vi "Periodic Tasks.vi"   [LabVIEW 2020]
doc: "This VI runs in parallel to other tasks. It can contain as many user-defined periodic loops as you need. These can carry out PID or other sorts of timed response."
uses:
  <vilib>/Rock Robotics/WPI/ThirdParty/JAS_Junk/TrajLib/PIDController_AtSetpoint.vi
  <vilib>/Rock Robotics/WPI/ThirdParty/JAS_Junk/TrajLib/PIDController_SetPIDF.vi
  <vilib>/Rock Robotics/WPI/ThirdParty/JAS_Junk/TrajLib/PIDController_SetDerivativeFilter.vi
  <vilib>/Rock Robotics/WPI/ThirdParty/JAS_Junk/TrajLib/PIDController_SetIntegratorRange.vi
  <vilib>/Rock Robotics/WPI/ThirdParty/JAS_Junk/TrajLib/PIDController_SetTolerancePandV.vi
  <vilib>/Rock Robotics/WPI/ThirdParty/JAS_Junk/TrajLib/PIDController_DisableContinousInput.vi
  <vilib>/Rock Robotics/WPI/ThirdParty/JAS_Junk/TrajLib/PIDController_EnableContinousInput.vi
  <vilib>/Rock Robotics/WPI/ThirdParty/JAS_Junk/TrajLib/PIDController_Reset.vi
  <vilib>/Rock Robotics/WPI/ThirdParty/JAS_Junk/TrajLib/PIDController_New.vi
  <vilib>/Rock Robotics/WPI/ThirdParty/JAS_Junk/TrajLib/PIDController_SetOutputLimits.vi
  <vilib>/Rock Robotics/WPI/ThirdParty/JAS_Junk/TrajLib/PIDController_NewPeriod.vi
  <vilib>/Rock Robotics/SystemInterfaces/NetworkCommunication/NetComm_UsageReport_report.vi
  Robot Global Data.vi
  <vilib>/Rock Robotics/WPI/ThirdParty/JAS_Junk/TrajLib/Util_LibraryGlobals.vi
  <vilib>/Rock Robotics/WPI/ThirdParty/JAS_Junk/TrajLib/PIDController_AdvCalculate_FF_Sp_Pv.vi
  <vilib>/Rock Robotics/WPI/ThirdParty/JAS_Junk/TrajLib/Trajectory_Library.lvlib
types:
  T1 = typedef "WPI_MotorControlDeviceRef.ctl" = cluster{"DeviceStatus":errorcluster, "Type":T2, "PWM":cluster{"PWM Channel":T3, "DeadBand":T4}, "CAN":cluster{"Device Number":u8, "SetOutput VI Ref":variant, "GetOutput VI Ref":variant, "Enable VI Ref":variant, "Disable VI Ref":variant, "Data":variant}, "Invert":bool, "DIO PWM":cluster{"PWM \"Enable\" Channel":T3, "DIOChannel":T5, "PWM Rate":dbl}}
  T2 = typedef "WPI_MotorControlType.ctl" = enum16{"PWM", "CAN", "DIO PWM"}
  T3 = typedef "FPGA_DIOPWMChannel.ctl" = enum8{"PWM 0", "PWM 1", "PWM 2", "PWM 3", "PWM 4", "PWM 5", "PWM 6", "PWM 7", "PWM 8", "PWM 9", "PWM MXP 0", "PWM MXP 1", "PWM MXP 2", "PWM MXP 3", "PWM MXP 4", "PWM MXP 5", "PWM MXP 6", "PWM MXP 7", "PWM MXP 8", "PWM MXP 9", "Invalid"}
  T4 = typedef "WPI_PWMDeadband.ctl" = cluster{"Name":string, "maxPositivePwm":i32, "minPositivePwm":i32, "centerPwm":i32, "maxNegativePwm":i32, "minNegativePwm":i32, "angularRange":u16}
  T5 = typedef "FPGA_DIOChannel.ctl" = enum8{"DIO 0", "DIO 1", "DIO 2", "DIO 3", "DIO 4", "DIO 5", "DIO 6", "DIO 7", "DIO 8", "DIO 9", "DIO MXP 0", "DIO MXP 1", "DIO MXP 2", "DIO MXP 3", "DIO MXP 4", "DIO MXP 5", "DIO MXP 6", "DIO MXP 7", "DIO MXP 8", "DIO MXP 9", "DIO MXP 10", "DIO MXP 11", "DIO MXP 12", "DIO MXP 13", "DIO MXP 14", "DIO MXP 15", "SPI Port CS1", "SPI Port CS2", "SPI Port CS3", "SPI Port MISO", "SPI Port MOSI", "Invalid"}
  T6 = typedef "WPI_GyroDevRef.ctl" = cluster{"DevStatus":errorcluster, "Analog Channel":T7, "Gain (VoltsPerDegree/Second)":dbl, "Gyro Type":enum16{"Analog", "XRS450"}, "Handle":i32, "SPI Bus":T8, "Device Found":bool, "Sample Rate":dbl, "Calibrate On Open":bool, "Offset":dbl}
  T7 = typedef "FPGA_AIChannel.ctl" = enum8{"AI 0", "AI 1", "AI 2", "AI 3", "AI MXP 0", "AI MXP 1", "AI MXP 2", "AI MXP 3", "Invalid"}
  T8 = typedef "spi_bus.ctl" = enum16{"SPI On-Board, CS0", "SPI On-Board, CS1", "SPI On-Board, CS2", "SPI On-Board, CS3", "SPI MXP", "Invalid"}
  T9 = typedef "Trajectory_Library.lvlib/ROTATION2D.ctl" = cluster{"VALUE":dbl, "COS":dbl, "SIN":dbl}
  T10 = typedef "Trajectory_Library.lvlib/SWERVE_DRIVE_MODULE_STATE.ctl" = cluster{"Speed":dbl, "Angle":T9}
  T11 = typedef "Trajectory_Library.lvlib/SWERVE_DRIVE_MODULE_POSITION.ctl" = cluster{"Distance":dbl, "Angle":T9, "P":bool}
  T12 = typedef "Trajectory_Library.lvlib/SWERVE_DRIVE_KINEMATICS.ctl" = cluster{"NumModules":i32, "InverseKinematics":T13, "ForwardKinematics":T13, "Modules":T14[], "PrevCoR":T14, "SavedModuleStates":T10[]}
  T13 = typedef "NI_Matrix.lvlib/RealMatrix.ctl" = dbl[][]
  T14 = typedef "Trajectory_Library.lvlib/TRANSLATION2D.ctl" = cluster{"X":dbl, "Y":dbl}
  T15 = typedef "Trajectory_Library.lvlib/SWERVE_DRIVE_ODOMETRY.ctl" = cluster{"POSE":T16, "GyroOffset":T9, "PreviousAngle":T9, "PrevModulePositions":T11[], "NumModules":i32}
  T16 = typedef "Trajectory_Library.lvlib/POSE2D.ctl" = cluster{"TRANSLATION":T14, "ROTATION":T9}
  T17 = cluster{"Max Input ":dbl, "Min Input ":dbl, "Continuous":bool, "Maximum Output":dbl, "Minimum Output ":dbl, "Kn":dbl, "KF":dbl, "KP":dbl, "KI":dbl, "KD":dbl, "Filter Derivative ":bool, "Max Integral":dbl, "Min Integral ":dbl}[]
  T18 = cluster{"Max Input ":dbl, "Min Input ":dbl, "Continuous":bool, "Maximum Output":dbl, "Minimum Output ":dbl, "Kn":dbl, "KF":dbl, "KP":dbl, "KI":dbl, "KD":dbl, "Filter Derivative ":bool, "Max Integral":dbl, "Min Integral ":dbl}
  T19 = typedef "Trajectory_Library.lvlib/PID_ADV_LIMITS.ctl" = cluster{"MaxInput":dbl, "MinInput":dbl, "Continuous":bool, "MaxOutput":dbl, "MinOutput":dbl}
  T20 = typedef "Trajectory_Library.lvlib/PID_ADV_TUNING.ctl" = cluster{"Kf":dbl, "Kp":dbl, "Ki":dbl, "Kd":dbl, "MaximumIntegral":dbl, "MinimumIntegral":dbl, "Filter Derivative":bool}
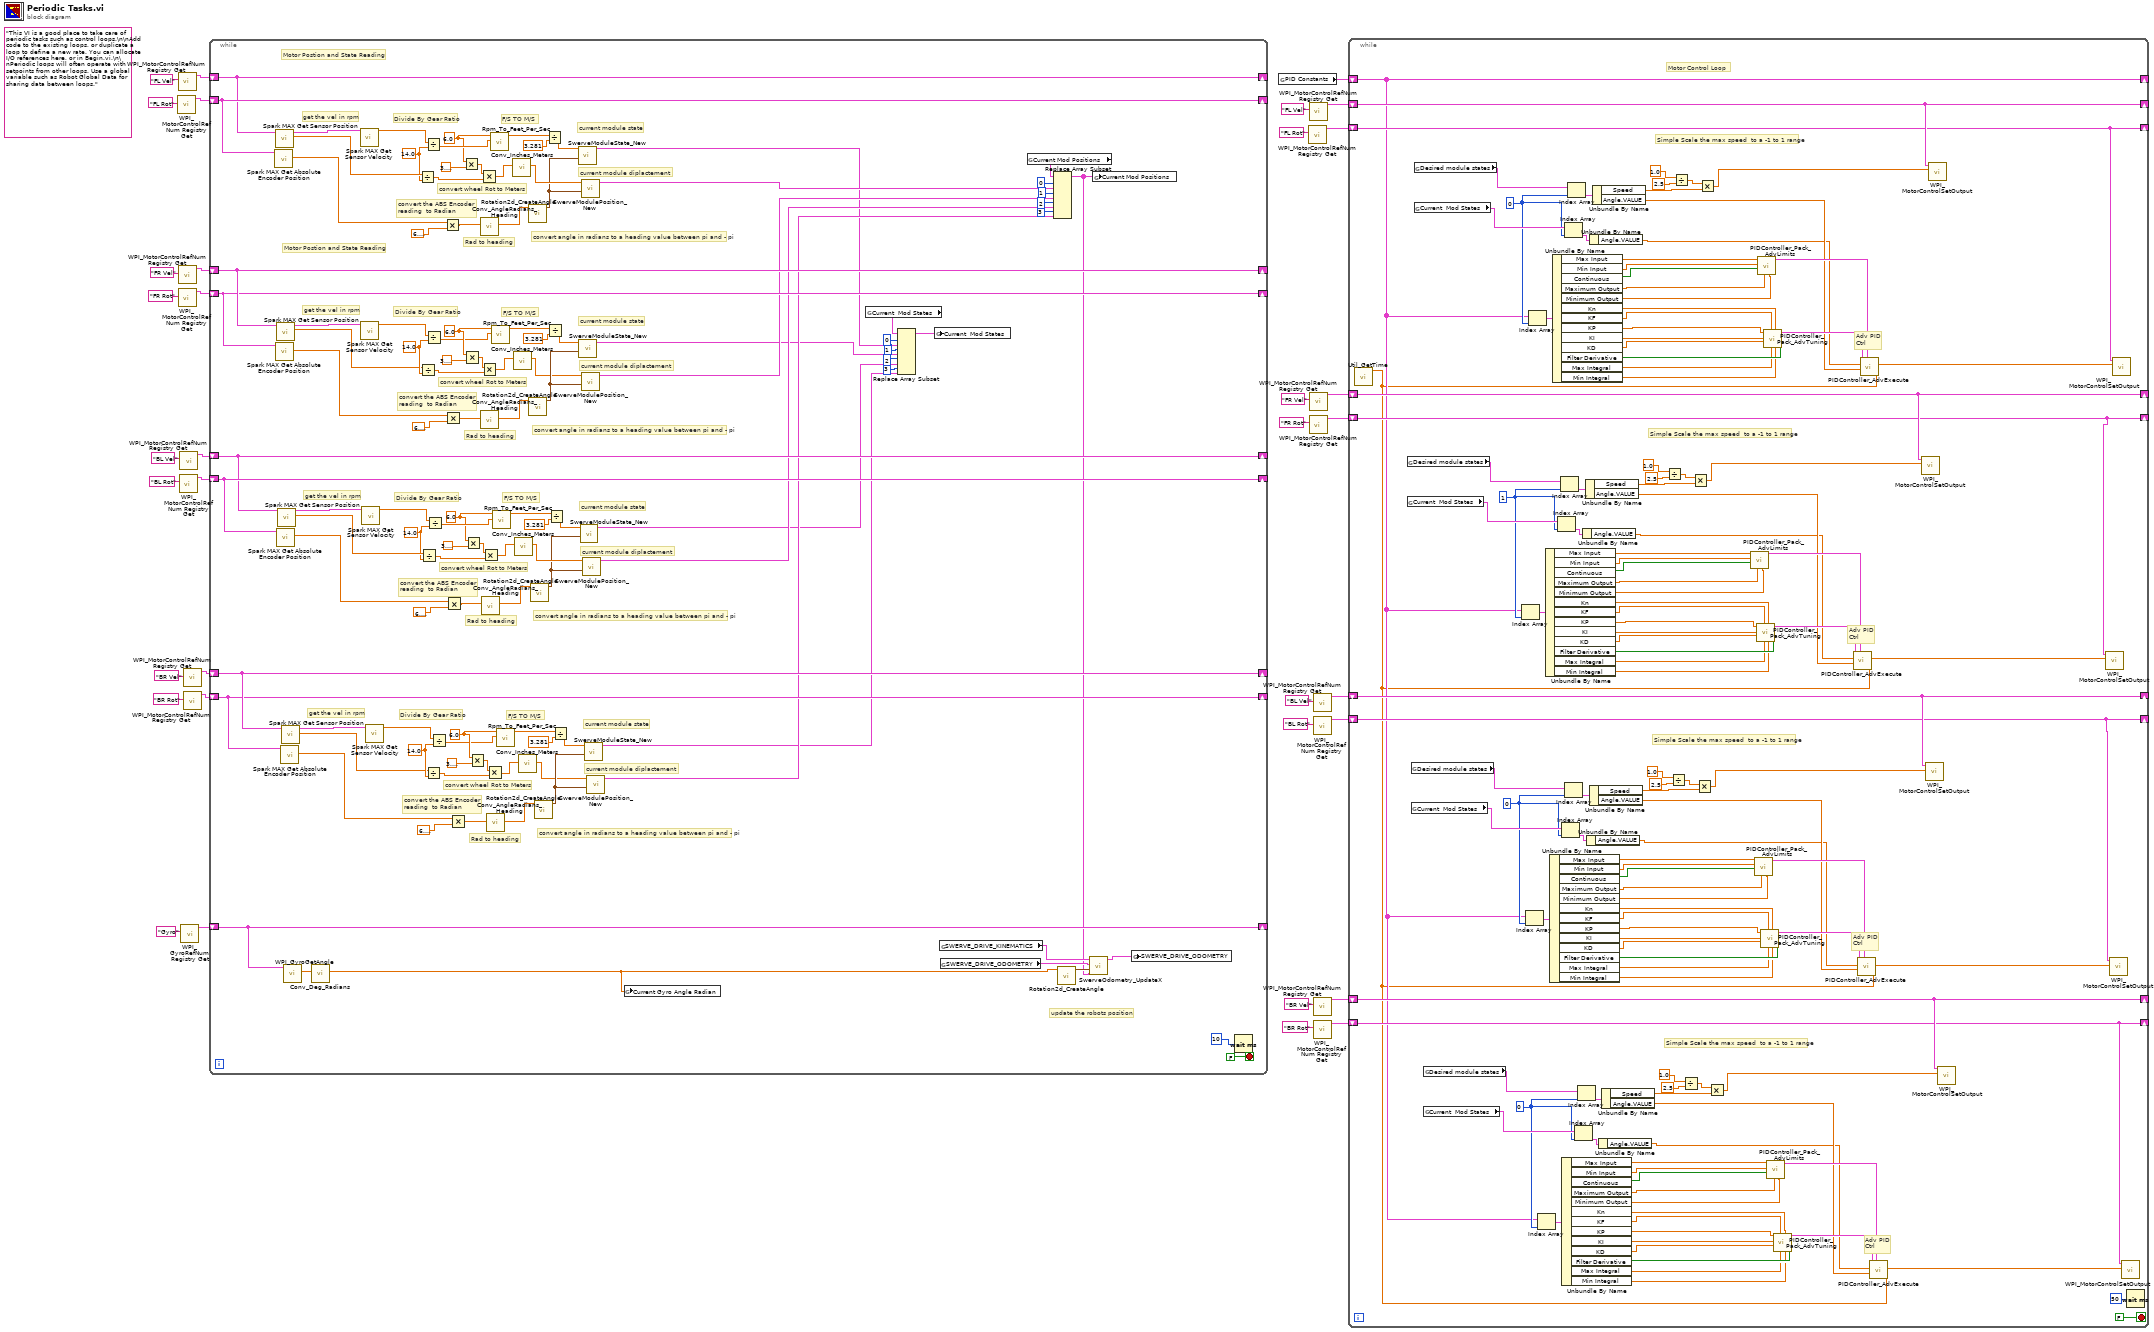
[diagram p0: block diagram]
diagram:
  (unwired) "This VI is a good place to take care of periodic tasks such as control loops.\n\nAdd code to the existing loops, or duplicate a loop to define a new rate. You can allocate I/O references here, or in Begin.vi.\n\nPeriodic loops will often operate with setpoints from other loops. Use a global variable such as Robot Global Data for sharing data between loops."
  n1 = call <vilib>:"WPI_MotorControlRefNum Registry Get.vi"("refnum name"="FL Rot") -> ("MotorControlDevRef"=w32:T1)  [unwired: 9 in, 1 out]
  n2 = call <vilib>:"WPI_MotorControlRefNum Registry Get.vi"("refnum name"="FL Vel") -> ("MotorControlDevRef"=w33:T1)  [unwired: 9 in, 1 out]
  n3 = call <vilib>:"WPI_MotorControlRefNum Registry Get.vi"("refnum name"="FR Rot") -> ("MotorControlDevRef"=w31:T1)  [unwired: 9 in, 1 out]
  n4 = call <vilib>:"WPI_MotorControlRefNum Registry Get.vi"("refnum name"="FR Vel") -> ("MotorControlDevRef"=w30:T1)  [unwired: 9 in, 1 out]
  n5 = call <vilib>:"WPI_MotorControlRefNum Registry Get.vi"("refnum name"="BL Rot") -> ("MotorControlDevRef"=w24:T1)  [unwired: 9 in, 1 out]
  n6 = call <vilib>:"WPI_MotorControlRefNum Registry Get.vi"("refnum name"="BL Vel") -> ("MotorControlDevRef"=w25:T1)  [unwired: 9 in, 1 out]
  n7 = call <vilib>:"WPI_GyroRefNum Registry Get.vi"("refnum name"="Gyro") -> ("GyroDevRef"=w1:T6)  [unwired: 9 in, 1 out]
  n8 = call <vilib>:"WPI_MotorControlRefNum Registry Get.vi"("refnum name"="BR Rot") -> ("MotorControlDevRef"=w23:T1)  [unwired: 9 in, 1 out]
  n9 = call <vilib>:"WPI_MotorControlRefNum Registry Get.vi"("refnum name"="BR Vel") -> ("MotorControlDevRef"=w22:T1)  [unwired: 9 in, 1 out]
  n10 = while {
    shift-right: [w126] -> _
    shift-left: w33 -> [w126]
    shift-right: [w127] -> _
    shift-left: w32 -> [w127]
    shift-right: [w125] -> _
    shift-left: w30 -> [w125]
    shift-right: [w124] -> _
    shift-left: w31 -> [w124]
    shift-right: [w84] -> _
    shift-left: w25 -> [w84]
    shift-right: [w85] -> _
    shift-left: w24 -> [w85]
    shift-right: [w83] -> _
    shift-left: w22 -> [w83]
    shift-right: [w82] -> _
    shift-left: w23 -> [w82]
    shift-right: [w38] -> _
    shift-left: w1 -> [w38]
    stop <- FALSE stop-if-true
    w80 = 14.0 ("y")
    w79 = 6.0 ("Diameter")
    w87 = 14.0 ("y")
    w88 = 6.0 ("Diameter")
    w122 = 14.0 ("y")
    w121 = 6.0 ("Diameter")
    w129 = 14.0 ("y")
    w130 = 6.0 ("Diameter")
    # "update the robots position"
    # "Rad to heading"
    # "convert wheel Rot to Meters"
    # "Divide By Gear Ratio"
    # "F/S TO M/S"
    # "current module diplactement"
    # "current module state"
    # "get the vel in rpm"
    # "convert angle in radians to a heading value between pi and - pi"
    # "convert the ABS Encoder \nreading  to Radian"
    # "Rad to heading"
    # "convert wheel Rot to Meters"
    # "Divide By Gear Ratio"
    # "F/S TO M/S"
    # "current module diplactement"
    # "current module state"
    # "get the vel in rpm"
    # "convert angle in radians to a heading value between pi and - pi"
    # "convert the ABS Encoder \nreading  to Radian"
    # "Rad to heading"
    # "convert wheel Rot to Meters"
    # "Divide By Gear Ratio"
    # "F/S TO M/S"
    # "current module diplactement"
    # "current module state"
    # "get the vel in rpm"
    # "convert angle in radians to a heading value between pi and - pi"
    # "convert the ABS Encoder \nreading  to Radian"
    # "Motor Postion and State Reading"
    # "Rad to heading"
    # "convert wheel Rot to Meters"
    # "Divide By Gear Ratio"
    # "F/S TO M/S"
    # "current module diplactement"
    # "current module state"
    # "get the vel in rpm"
    # "convert angle in radians to a heading value between pi and - pi"
    # "convert the ABS Encoder \nreading  to Radian"
    # "Motor Postion and State Reading"
    n11 = call <vilib>:"Spark MAX Get Absolute Encoder Position.vi"("MotorControlDeviceRef in"=w127) -> ("Position"=w145:dbl)  [unwired: 7 in, 3 out]
    n12 = call <vilib>:"Spark MAX Get Sensor Position.vi"("MotorControlDevRef in"=w126) -> ("Sensor Position"=w140:dbl, "MotorControlDevRef out"=w135:T1)  [unwired: 7 in, 2 out]
    n13 = call <vilib>:"Spark MAX Get Absolute Encoder Position.vi"("MotorControlDeviceRef in"=w124) -> ("Position"=w106:dbl)  [unwired: 7 in, 3 out]
    n14 = call <vilib>:"Spark MAX Get Sensor Position.vi"("MotorControlDevRef in"=w125) -> ("Sensor Position"=w111:dbl, "MotorControlDevRef out"=w116:T1)  [unwired: 7 in, 2 out]
    n15 = call <vilib>:"Spark MAX Get Absolute Encoder Position.vi"("MotorControlDeviceRef in"=w85) -> ("Position"=w103:dbl)  [unwired: 7 in, 3 out]
    n16 = call <vilib>:"Spark MAX Get Sensor Position.vi"("MotorControlDevRef in"=w84) -> ("Sensor Position"=w98:dbl, "MotorControlDevRef out"=w93:T1)  [unwired: 7 in, 2 out]
    n17 = call <vilib>:"Spark MAX Get Absolute Encoder Position.vi"("MotorControlDeviceRef in"=w82) -> ("Position"=w64:dbl)  [unwired: 7 in, 3 out]
    n18 = call <vilib>:"Spark MAX Get Sensor Position.vi"("MotorControlDevRef in"=w83) -> ("Sensor Position"=w69:dbl, "MotorControlDevRef out"=w74:T1)  [unwired: 7 in, 2 out]
    n19 = call <vilib>:"WPI_GyroGetAngle.vi"("GyroDevRef"=w38) -> ("Angle"=w42:dbl)  [unwired: 6 in, 4 out]
    n20 = call <vilib>:"Conv_Deg_Radians.vi"("Degress"=w42) -> ("Radians"=w36:dbl)  [unwired: 10 in]
    n21 = call <vilib>:"Spark MAX Get Sensor Velocity.vi"("MotorControlDevRef in"=w135) -> ("Sensor Velocity"=w137:dbl)  [unwired: 7 in, 3 out]
    n22 = call <vilib>:"Spark MAX Get Sensor Velocity.vi"("MotorControlDevRef in"=w116) -> ("Sensor Velocity"=w114:dbl)  [unwired: 7 in, 3 out]
    n23 = call <vilib>:"Spark MAX Get Sensor Velocity.vi"("MotorControlDevRef in"=w93) -> ("Sensor Velocity"=w95:dbl)  [unwired: 7 in, 3 out]
    n24 = call <vilib>:"Spark MAX Get Sensor Velocity.vi"("MotorControlDevRef in"=w74) -> ("Sensor Velocity"=w72:dbl)  [unwired: 7 in, 3 out]
    n25 = Divide(x=w140, y=w129) -> (x/y=w143:dbl)
    n26 = Divide(x=w111, y=w122) -> (x/y=w108:dbl)
    n27 = Divide(x=w98, y=w87) -> (x/y=w101:dbl)
    n28 = Divide(x=w137, y=w129) -> (x/y=w139:dbl)
    n29 = Divide(x=w69, y=w80) -> (x/y=w66:dbl)
    n30 = Divide(x=w114, y=w122) -> (x/y=w112:dbl)
    n31 = Divide(x=w95, y=w87) -> (x/y=w97:dbl)
    n32 = Divide(x=w72, y=w80) -> (x/y=w70:dbl)
    n33 = Multiply(x=w145, y=6.283185307179586) -> (x*y=w146:dbl)
    n34 = Multiply(x=w106, y=6.283185307179586) -> (x*y=w105:dbl)
    n35 = Multiply(x=w103, y=6.283185307179586) -> (x*y=w104:dbl)
    n36 = Multiply(x=w64, y=6.283185307179586) -> (x*y=w63:dbl)
    n37 = Multiply(x=w130, y=3.141592653589793) -> (x*y=w142:dbl)
    n38 = Multiply(x=w121, y=3.141592653589793) -> (x*y=w109:dbl)
    n39 = Multiply(x=w88, y=3.141592653589793) -> (x*y=w100:dbl)
    n40 = Multiply(x=w79, y=3.141592653589793) -> (x*y=w67:dbl)
    n41 = Multiply(x=w142, y=w143) -> (x*y=w141:dbl)
    n42 = call <vilib>:"Conv_AngleRadians_Heading.vi"("Radians"=w146) -> ("Heading"=w134:dbl)  [unwired: 10 in]
    n43 = Multiply(x=w109, y=w108) -> (x*y=w110:dbl)
    n44 = call <vilib>:"Conv_AngleRadians_Heading.vi"("Radians"=w105) -> ("Heading"=w117:dbl)  [unwired: 10 in]
    n45 = Multiply(x=w100, y=w101) -> (x*y=w99:dbl)
    n46 = call <vilib>:"Conv_AngleRadians_Heading.vi"("Radians"=w104) -> ("Heading"=w92:dbl)  [unwired: 10 in]
    n47 = Multiply(x=w67, y=w66) -> (x*y=w68:dbl)
    n48 = call <vilib>:"Conv_AngleRadians_Heading.vi"("Radians"=w63) -> ("Heading"=w75:dbl)  [unwired: 10 in]
    n49 = call "Rpm_To_Feet_Per_Sec.vi"("RPM"=w139, "Diameter"=w130) -> ("Numeric"=w138:dbl)  [unwired: 9 in]
    n50 = call "Rpm_To_Feet_Per_Sec.vi"("RPM"=w112, "Diameter"=w121) -> ("Numeric"=w113:dbl)  [unwired: 9 in]
    n51 = call "Rpm_To_Feet_Per_Sec.vi"("RPM"=w97, "Diameter"=w88) -> ("Numeric"=w96:dbl)  [unwired: 9 in]
    n52 = call "Rpm_To_Feet_Per_Sec.vi"("RPM"=w70, "Diameter"=w79) -> ("Numeric"=w71:dbl)  [unwired: 9 in]
    n53 = call <vilib>:"Conv_Inches_Meters.vi"("INCH"=w141) -> ("Meters"=w144:dbl)  [unwired: 10 in]
    n54 = call <vilib>:"Conv_Inches_Meters.vi"("INCH"=w110) -> ("Meters"=w107:dbl)  [unwired: 10 in]
    n55 = call <vilib>:"Conv_Inches_Meters.vi"("INCH"=w99) -> ("Meters"=w102:dbl)  [unwired: 10 in]
    n56 = call <vilib>:"Conv_Inches_Meters.vi"("INCH"=w68) -> ("Meters"=w65:dbl)  [unwired: 10 in]
    n57 = call <vilib>:"Rotation2d_CreateAngle.vi"("Angle"=w134) -> ("ROTATION"=w133:T9)  [unwired: 10 in]
    n58 = call <vilib>:"Rotation2d_CreateAngle.vi"("Angle"=w117) -> ("ROTATION"=w118:T9)  [unwired: 10 in]
    n59 = call <vilib>:"Rotation2d_CreateAngle.vi"("Angle"=w92) -> ("ROTATION"=w91:T9)  [unwired: 10 in]
    n60 = call <vilib>:"Rotation2d_CreateAngle.vi"("Angle"=w75) -> ("ROTATION"=w76:T9)  [unwired: 10 in]
    n61 = Divide(x=w138, y=3.281) -> (x/y=w136:dbl)
    n62 = Divide(x=w113, y=3.281) -> (x/y=w115:dbl)
    n63 = Divide(x=w96, y=3.281) -> (x/y=w94:dbl)
    n64 = Divide(x=w71, y=3.281) -> (x/y=w73:dbl)
    n65 = call <vilib>:"SwerveModuleState_New.vi"("ROTATION"=w133, "Speed"=w136) -> ("SWERVE_DRIVE_MODULE_STATE"=w48:T10)  [unwired: 9 in]
    n66 = call <vilib>:"SwerveModuleState_New.vi"("ROTATION"=w118, "Speed"=w115) -> ("SWERVE_DRIVE_MODULE_STATE"=w47:T10)  [unwired: 9 in]
    n67 = call <vilib>:"SwerveModuleState_New.vi"("ROTATION"=w91, "Speed"=w94) -> ("SWERVE_DRIVE_MODULE_STATE"=w46:T10)  [unwired: 9 in]
    n68 = call <vilib>:"SwerveModulePosition_New.vi"("ROTATION"=w133, "Distance"=w144) -> ("SWERVE_DRIVE_MODULE_POSITION"=w57:T11)  [unwired: 9 in]
    n69 = call <vilib>:"SwerveModulePosition_New.vi"("ROTATION"=w118, "Distance"=w107) -> ("SWERVE_DRIVE_MODULE_POSITION"=w56:T11)  [unwired: 9 in]
    n70 = call <vilib>:"SwerveModulePosition_New.vi"("ROTATION"=w91, "Distance"=w102) -> ("SWERVE_DRIVE_MODULE_POSITION"=w55:T11)  [unwired: 9 in]
    n71 = call <vilib>:"SwerveModuleState_New.vi"("ROTATION"=w76, "Speed"=w73) -> ("SWERVE_DRIVE_MODULE_STATE"=w45:T10)  [unwired: 9 in]
    n72 = call <vilib>:"SwerveModulePosition_New.vi"("ROTATION"=w76, "Distance"=w65) -> ("SWERVE_DRIVE_MODULE_POSITION"=w54:T11)  [unwired: 9 in]
    n73 = global write "Robot Global Data.vi" "Current Gyro Angle Radian"(w36) -> ()
    n74 = global read "Robot Global Data.vi" "Current  Mod States"() -> (w53:T10[])
    n75 = Replace Array Subset(array=w53, new element #1=w48, index #1=0 ("index"), new element #2=w47, index #2=1 ("index"), new element #3=w46, index #3=2 ("index"), new element #4=w45, index #4=3 ("index")) -> (w44:T10[])
    n76 = global write "Robot Global Data.vi" "Current  Mod States"(w44) -> ()
    n77 = global read "Robot Global Data.vi" "SWERVE_DRIVE_KINEMATICS"() -> (w40:T12)
    n78 = global read "Robot Global Data.vi" "SWERVE_DRIVE_ODOMETRY"() -> (w41:T15)
    n79 = global read "Robot Global Data.vi" "Current Mod Positions"() -> (w58:T11[])
    n80 = Replace Array Subset(array=w58, new element #1=w57, index #1=0 ("index"), new element #2=w56, index #2=1 ("index"), new element #3=w55, index #3=2 ("index"), new element #4=w54, index #4=3 ("index")) -> (w37:T11[])
    n81 = call <vilib>:"Rotation2d_CreateAngle.vi"("Angle"=w36) -> ("ROTATION"=w39:T9)  [unwired: 10 in]
    n82 = call <vilib>:"SwerveOdometry_UpdateX.vi"("module Positions"=w37, "gyroAngle"=w39, "in SWERVE_DRIVE_ODOMETRY"=w41, "SWERVE_DRIVE_KINEMATICS"=w40) -> ("out SWERVE_DRIVE_ODOMETRY"=w43:T15)  [unwired: 5 in, 2 out]
    n83 = global write "Robot Global Data.vi" "Current Mod Positions"(w37) -> ()
    n84 = global write "Robot Global Data.vi" "SWERVE_DRIVE_ODOMETRY"(w43) -> ()
    n85 = Wait (ms)(milliseconds to wait=u32 10) -> ()  [unwired: 1 out]
  }
  n86 = global read "Robot Global Data.vi" "PID Constants"() -> (w3:T17)
  n87 = call <vilib>:"WPI_MotorControlRefNum Registry Get.vi"("refnum name"="FL Rot") -> ("MotorControlDevRef"=w10:T1)  [unwired: 9 in, 1 out]
  n88 = call <vilib>:"WPI_MotorControlRefNum Registry Get.vi"("refnum name"="FL Vel") -> ("MotorControlDevRef"=w11:T1)  [unwired: 9 in, 1 out]
  n89 = call <vilib>:"WPI_MotorControlRefNum Registry Get.vi"("refnum name"="FR Rot") -> ("MotorControlDevRef"=w8:T1)  [unwired: 9 in, 1 out]
  n90 = call <vilib>:"WPI_MotorControlRefNum Registry Get.vi"("refnum name"="FR Vel") -> ("MotorControlDevRef"=w9:T1)  [unwired: 9 in, 1 out]
  n91 = call <vilib>:"WPI_MotorControlRefNum Registry Get.vi"("refnum name"="BL Rot") -> ("MotorControlDevRef"=w6:T1)  [unwired: 9 in, 1 out]
  n92 = call <vilib>:"WPI_MotorControlRefNum Registry Get.vi"("refnum name"="BR Rot") -> ("MotorControlDevRef"=w4:T1)  [unwired: 9 in, 1 out]
  n93 = call <vilib>:"WPI_MotorControlRefNum Registry Get.vi"("refnum name"="BL Vel") -> ("MotorControlDevRef"=w7:T1)  [unwired: 9 in, 1 out]
  n94 = call <vilib>:"WPI_MotorControlRefNum Registry Get.vi"("refnum name"="BR Vel") -> ("MotorControlDevRef"=w5:T1)  [unwired: 9 in, 1 out]
  n95 = while {
    shift-right: [w247] -> _
    shift-left: w11 -> [w247]
    shift-right: [w244] -> _
    shift-left: w10 -> [w244]
    shift-right: [w214] -> _
    shift-left: w9 -> [w214]
    shift-right: [w213] -> _
    shift-left: w8 -> [w213]
    shift-right: [w183] -> _
    shift-left: w7 -> [w183]
    shift-right: [w182] -> _
    shift-left: w6 -> [w182]
    shift-right: [w152] -> _
    shift-left: w5 -> [w152]
    shift-right: [w151] -> _
    shift-left: w4 -> [w151]
    shift-right: [w150] -> _
    shift-left: w3 -> [w150]
    stop <- FALSE stop-if-true
    w155 = 0 ("index")
    w186 = 0 ("index")
    w217 = 1 ("index")
    w248 = 0 ("index")
    # "Simple Scale the max speed  to a -1 to 1 range"
    # "Adv PID\nCtrl"
    # "Simple Scale the max speed  to a -1 to 1 range"
    # "Adv PID\nCtrl"
    # "Simple Scale the max speed  to a -1 to 1 range"
    # "Adv PID\nCtrl"
    # "Simple Scale the max speed  to a -1 to 1 range"
    # "Adv PID\nCtrl"
    # "Motor Control Loop"
    n96 = call <vilib>:"Util_GetTime.vi"() -> ("FPGA_Time_Seconds"=w149:dbl)  [unwired: 9 in, 2 out]
    n97 = global read "Robot Global Data.vi" "Desired module states"() -> (w240:T10[])
    n98 = global read "Robot Global Data.vi" "Current  Mod States"() -> (w236:T10[])
    n99 = global read "Robot Global Data.vi" "Desired module states"() -> (w209:T10[])
    n100 = global read "Robot Global Data.vi" "Current  Mod States"() -> (w205:T10[])
    n101 = global read "Robot Global Data.vi" "Desired module states"() -> (w271:T10[])
    n102 = global read "Robot Global Data.vi" "Current  Mod States"() -> (w267:T10[])
    n103 = global read "Robot Global Data.vi" "Desired module states"() -> (w178:T10[])
    n104 = global read "Robot Global Data.vi" "Current  Mod States"() -> (w174:T10[])
    n105 = Index Array(array=w150, index=w217) -> (element=w233:T18)
    n106 = Index Array(array=w150, index=w186) -> (element=w202:T18)
    n107 = Index Array(array=w150, index=w248) -> (element=w264:T18)
    n108 = Index Array(array=w150, index=w155) -> (element=w171:T18)
    n109 = Unbundle By Name(w233) -> ("Max Input"=w232:dbl, "Min Input"=w231:dbl, "Continuous"=w230:bool, "Maximum Output"=w229:dbl, "Minimum Output"=w228:dbl, "Kn"=w227:dbl, "KF"=w226:dbl, "KP"=w225:dbl, "KI"=w224:dbl, "KD"=w223:dbl, "Filter Derivative"=w222:bool, "Max Integral"=w221:dbl, "Min Integral"=w220:dbl)
    n110 = Unbundle By Name(w202) -> ("Max Input"=w201:dbl, "Min Input"=w200:dbl, "Continuous"=w199:bool, "Maximum Output"=w198:dbl, "Minimum Output"=w197:dbl, "Kn"=w196:dbl, "KF"=w195:dbl, "KP"=w194:dbl, "KI"=w193:dbl, "KD"=w192:dbl, "Filter Derivative"=w191:bool, "Max Integral"=w190:dbl, "Min Integral"=w189:dbl)
    n111 = Unbundle By Name(w264) -> ("Max Input"=w263:dbl, "Min Input"=w262:dbl, "Continuous"=w261:bool, "Maximum Output"=w260:dbl, "Minimum Output"=w259:dbl, "Kn"=w258:dbl, "KF"=w257:dbl, "KP"=w256:dbl, "KI"=w255:dbl, "KD"=w254:dbl, "Filter Derivative"=w253:bool, "Max Integral"=w252:dbl, "Min Integral"=w251:dbl)
    n112 = Index Array(array=w236, index=w217) -> (element=w237:T10)
    n113 = Index Array(array=w240, index=w217) -> (element=w239:T10)
    n114 = Index Array(array=w205, index=w186) -> (element=w206:T10)
    n115 = Unbundle By Name(w171) -> ("Max Input"=w170:dbl, "Min Input"=w169:dbl, "Continuous"=w168:bool, "Maximum Output"=w167:dbl, "Minimum Output"=w166:dbl, "Kn"=w165:dbl, "KF"=w164:dbl, "KP"=w163:dbl, "KI"=w162:dbl, "KD"=w161:dbl, "Filter Derivative"=w160:bool, "Max Integral"=w159:dbl, "Min Integral"=w158:dbl)
    n116 = Index Array(array=w267, index=w248) -> (element=w268:T10)
    n117 = Index Array(array=w209, index=w186) -> (element=w208:T10)
    n118 = Index Array(array=w271, index=w248) -> (element=w270:T10)
    n119 = Index Array(array=w174, index=w155) -> (element=w175:T10)
    n120 = Index Array(array=w178, index=w155) -> (element=w177:T10)
    n121 = Unbundle By Name(w237) -> ("Angle.VALUE"=w218:dbl)
    n122 = Unbundle By Name(w239) -> ("Speed"=w238:dbl, "Angle.VALUE"=w219:dbl)
    n123 = Unbundle By Name(w206) -> ("Angle.VALUE"=w187:dbl)
    n124 = Unbundle By Name(w268) -> ("Angle.VALUE"=w249:dbl)
    n125 = Unbundle By Name(w208) -> ("Speed"=w207:dbl, "Angle.VALUE"=w188:dbl)
    n126 = Unbundle By Name(w270) -> ("Speed"=w269:dbl, "Angle.VALUE"=w250:dbl)
    n127 = Unbundle By Name(w175) -> ("Angle.VALUE"=w156:dbl)
    n128 = Unbundle By Name(w177) -> ("Speed"=w176:dbl, "Angle.VALUE"=w157:dbl)
    n129 = Divide(x=1.0, y=2.5) -> (x/y=w241:dbl)
    n130 = Divide(x=1.0, y=2.5) -> (x/y=w210:dbl)
    n131 = Divide(x=1.0, y=2.5) -> (x/y=w272:dbl)
    n132 = Divide(x=1.0, y=2.5) -> (x/y=w179:dbl)
    n133 = Multiply(x=w241, y=w238) -> (x*y=w216:dbl)
    n134 = Multiply(x=w210, y=w207) -> (x*y=w185:dbl)
    n135 = Multiply(x=w272, y=w269) -> (x*y=w246:dbl)
    n136 = Multiply(x=w179, y=w176) -> (x*y=w154:dbl)
    n137 = call <vilib>:"PIDController_Pack_AdvLimits.vi"("MinOutput"=w228, "MaxOutput"=w229, "Continuous"=w230, "MinInput"=w231, "MaxInput"=w232) -> ("Adv PID Limits"=w234:T19)  [unwired: 6 in]
    n138 = call <vilib>:"PIDController_Pack_AdvLimits.vi"("MinOutput"=w197, "MaxOutput"=w198, "Continuous"=w199, "MinInput"=w200, "MaxInput"=w201) -> ("Adv PID Limits"=w203:T19)  [unwired: 6 in]
    n139 = call <vilib>:"PIDController_Pack_AdvTuning.vi"("Filter Derivative"=w222, "MinimumIntegral"=w220, "Kn"=w227, "MaximumIntegral"=w221, "Kf"=w226, "Kd"=w223, "Ki"=w224, "Kp"=w225) -> ("Adv PID Tuning"=w235:T20)  [unwired: 3 in]
    n140 = call <vilib>:"PIDController_Pack_AdvLimits.vi"("MinOutput"=w259, "MaxOutput"=w260, "Continuous"=w261, "MinInput"=w262, "MaxInput"=w263) -> ("Adv PID Limits"=w265:T19)  [unwired: 6 in]
    n141 = call <vilib>:"PIDController_Pack_AdvTuning.vi"("Filter Derivative"=w191, "MinimumIntegral"=w189, "Kn"=w196, "MaximumIntegral"=w190, "Kf"=w195, "Kd"=w192, "Ki"=w193, "Kp"=w194) -> ("Adv PID Tuning"=w204:T20)  [unwired: 3 in]
    n142 = call <vilib>:"PIDController_Pack_AdvTuning.vi"("Filter Derivative"=w253, "MinimumIntegral"=w251, "Kn"=w258, "MaximumIntegral"=w252, "Kf"=w257, "Kd"=w254, "Ki"=w255, "Kp"=w256) -> ("Adv PID Tuning"=w266:T20)  [unwired: 3 in]
    n143 = call <vilib>:"PIDController_Pack_AdvLimits.vi"("MinOutput"=w166, "MaxOutput"=w167, "Continuous"=w168, "MinInput"=w169, "MaxInput"=w170) -> ("Adv PID Limits"=w172:T19)  [unwired: 6 in]
    n144 = call <vilib>:"PIDController_Pack_AdvTuning.vi"("Filter Derivative"=w160, "MinimumIntegral"=w158, "Kn"=w165, "MaximumIntegral"=w159, "Kf"=w164, "Kd"=w161, "Ki"=w162, "Kp"=w163) -> ("Adv PID Tuning"=w173:T20)  [unwired: 3 in]
    n145 = call <vilib>:"PIDController_AdvExecute.vi"("Time"=w149, "Adv PID Limits"=w234, "SP-SetPoint"=w219, "PV-Measurement"=w218, "Adv PID Tuning"=w235) -> ("CO-ControlOutput"=w215:dbl)  [unwired: 4 in, 2 out]
    n146 = call <vilib>:"PIDController_AdvExecute.vi"("Time"=w149, "Adv PID Limits"=w203, "SP-SetPoint"=w188, "PV-Measurement"=w187, "Adv PID Tuning"=w204) -> ("CO-ControlOutput"=w184:dbl)  [unwired: 4 in, 2 out]
    n147 = call <vilib>:"PIDController_AdvExecute.vi"("Time"=w149, "Adv PID Limits"=w265, "SP-SetPoint"=w250, "PV-Measurement"=w249, "Adv PID Tuning"=w266) -> ("CO-ControlOutput"=w245:dbl)  [unwired: 4 in, 2 out]
    n148 = call <vilib>:"PIDController_AdvExecute.vi"("Time"=w149, "Adv PID Limits"=w172, "SP-SetPoint"=w157, "PV-Measurement"=w156, "Adv PID Tuning"=w173) -> ("CO-ControlOutput"=w153:dbl)  [unwired: 4 in, 2 out]
    n149 = call <vilib>:"WPI_MotorControlSetOutput.vi"("Output"=w216, "MotorControlDevRef"=w214) -> ()  [unwired: 7 in, 3 out]
    n150 = call <vilib>:"WPI_MotorControlSetOutput.vi"("Output"=w185, "MotorControlDevRef"=w183) -> ()  [unwired: 7 in, 3 out]
    n151 = call <vilib>:"WPI_MotorControlSetOutput.vi"("Output"=w246, "MotorControlDevRef"=w247) -> ()  [unwired: 7 in, 3 out]
    n152 = call <vilib>:"WPI_MotorControlSetOutput.vi"("Output"=w154, "MotorControlDevRef"=w152) -> ()  [unwired: 7 in, 3 out]
    n153 = call <vilib>:"WPI_MotorControlSetOutput.vi"("Output"=w215, "MotorControlDevRef"=w213) -> ()  [unwired: 7 in, 3 out]
    n154 = call <vilib>:"WPI_MotorControlSetOutput.vi"("Output"=w184, "MotorControlDevRef"=w182) -> ()  [unwired: 7 in, 3 out]
    n155 = call <vilib>:"WPI_MotorControlSetOutput.vi"("Output"=w245, "MotorControlDevRef"=w244) -> ()  [unwired: 7 in, 3 out]
    n156 = call <vilib>:"WPI_MotorControlSetOutput.vi"("Output"=w153, "MotorControlDevRef"=w151) -> ()  [unwired: 7 in, 3 out]
    n157 = Wait (ms)(milliseconds to wait=u32 50) -> ()  [unwired: 1 out]
  }
